vi "lib 699 Mission Telem Filename.vi"(4 "Mission":string) -> (1 "TM File":string)   [LabVIEW 2014]
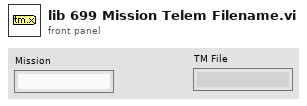
[diagram p1: front panel]
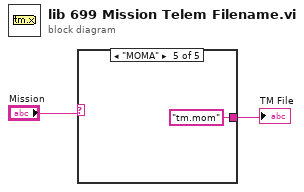
[diagram p0: block diagram]
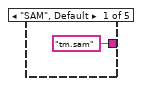
[diagram p2: hidden frame]
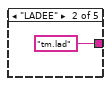
[diagram p3: hidden frame]
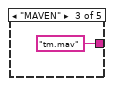
[diagram p4: hidden frame]
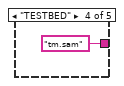
[diagram p5: hidden frame]
diagram:
  n1 = case shown="\"MOMA\"" "Mission" {
    tunnel: ["tm.sam" "tm.lad" "tm.mav" "tm.sam" "tm.mom"] -> w1
    frame "SAM", Default {
    }
    frame "LADEE" {
    }
    frame "MAVEN" {
    }
    frame "TESTBED" {
    }
    frame "MOMA" {
    }
  }
  "TM File" <- w1
